vi "Get Array of HWplugin Objs.vi"(8 "error in (no error)":errorcluster, 10 "HW type":string, 11 "Function in":refnum<class "Function.lvclass">) -> (0 "error out":errorcluster, 1 "found":bool, 2 "Array of HWplugin Objs":refnum<class "Hardware.lvclass">[](array[class]), 3 "Function out":refnum<class "Function.lvclass">)   [LabVIEW 2016, in "Function Actor.lvlib" / "Function.lvclass"]
uses:
  <userlib>/Common Components/Function Actor/Function.lvclass
  <userlib>/Common Components/Hardware/Abstract Hardware/Hardware.lvclass
  <userlib>/Common Components/Function Actor/Function.lvclass/Function.ctl
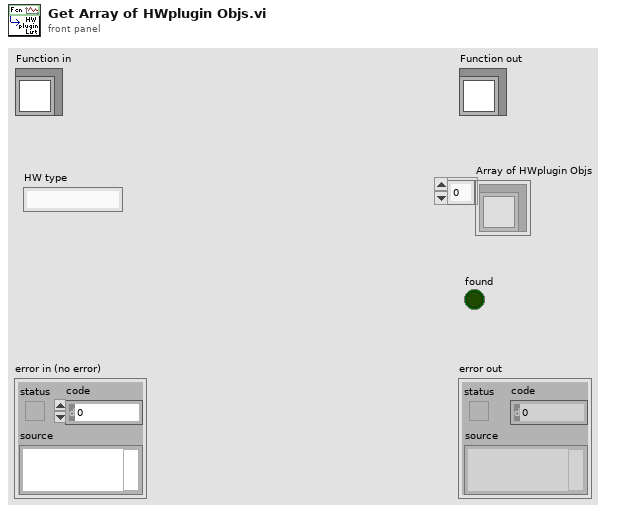
[diagram p1: front panel]
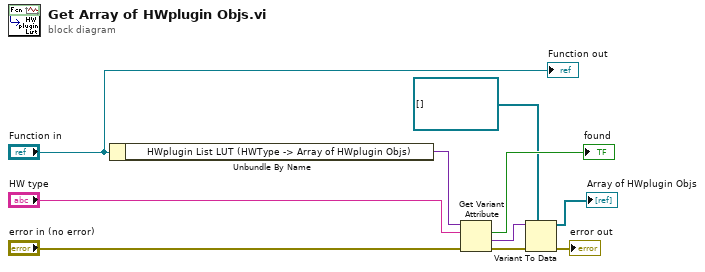
[diagram p0: block diagram]
diagram:
  n1 = Unbundle By Name("Function in") -> ("HWplugin List LUT (HWType -> Array of HWplugin Objs)"=w9:variant)
  n2 = Get Variant Attribute(Variant=w9, name="HW type", error in="error in (no error)") -> (found=→"found":bool, value=w7:variant, error out=w3:errorcluster)  [unwired: 1 in, 1 out]
  n3 = Variant To Data(error in=w3, type=refnum<class "Hardware.lvclass">[] [], Variant=w7) -> (data=→"Array of HWplugin Objs":refnum<class "Hardware.lvclass">[], error out=→"error out":errorcluster)
  "Function out" <- "Function in"
